vi "IncOpCount.vi"(9 "inc?":bool, 11 "MessengerMCPU in":refnum<class "MessengerMCPU.lvclass">) -> (3 "MessengerMCPU out":refnum<class "MessengerMCPU.lvclass">)   [LabVIEW 2019, in "MessengerM.lvlib" / "MessengerMCPU.lvclass"]
uses:
  MessengerMCPU.lvclass
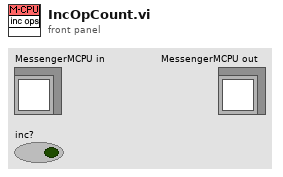
[diagram p1: front panel]
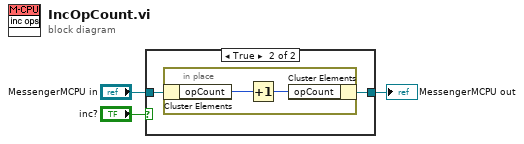
[diagram p0: block diagram]
diagram:
  n1 = case shown="True" "inc?" {
    tunnel: "MessengerMCPU in" -> [w4 w6]
    tunnel: [w4 w5] -> w2
    frame False {
    }
    frame True {
      n2 = in-place {
        n3 = in-place-cluster #1(w6) -> ("opCount"=w8:u32)
        n4 = Increment(x=w8) -> (x+1=w7:u32)
        n5 = in-place-cluster #1("opCount"=w7) -> (w5:refnum<class "MessengerMCPU.lvclass">)
      }
    }
  }
  "MessengerMCPU out" <- w2
